vi "build token URI.vi"(8 "error in (no error)":errorcluster, 11 "Oauth2.Google in":refnum<class "Oauth2.Google.lvclass">) -> (0 "error out":errorcluster, 1 "Headers":cluster{"header":string, "value":string}[](array[cluster]), 2 "Token Request URI":string, 3 "Oauth2.Google":refnum<class "Oauth2.Google.lvclass">)   [LabVIEW 2013, in "Oauth2.Google.lvclass"]
uses:
  Oauth2.Google.lvclass
  OAuthToken/OAuth2 Token Element -- enum.ctl
  Oauth2.Google.lvclass/Oauth2.Google.ctl
  <vilib>/LabVIEW Open Source Project/OpenURI/uri/URI.lvclass
  OAuthToken/OAuthAccessToken.lvclass
  Oauth2/Oauth2.lvclass
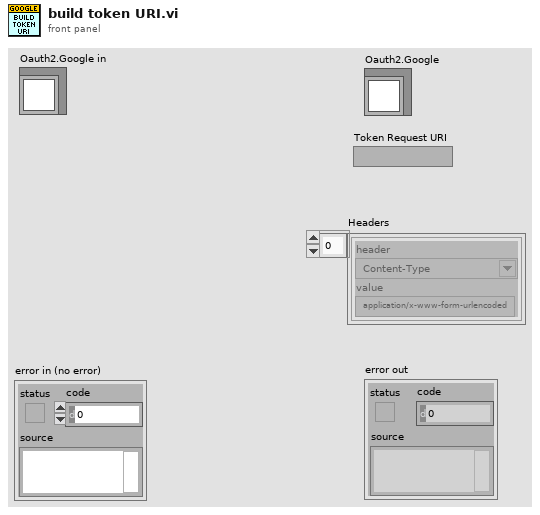
[diagram p1: front panel]
types:
  T1 = typedef "OAuthAccessToken.lvclass/OAuth2 Token Element -- enum.ctl" = enum16{"client_id", "client_secret", "response_type", "scope", "redirect_uri", "error", "error_description", "error_uri", "grant_type", "code", "access_token", "token_type", "expires_in", "username", "password", "refresh_token", "code_challenge", "code_challenge_method", "reverse_proxy_uri", "endpoint element"}
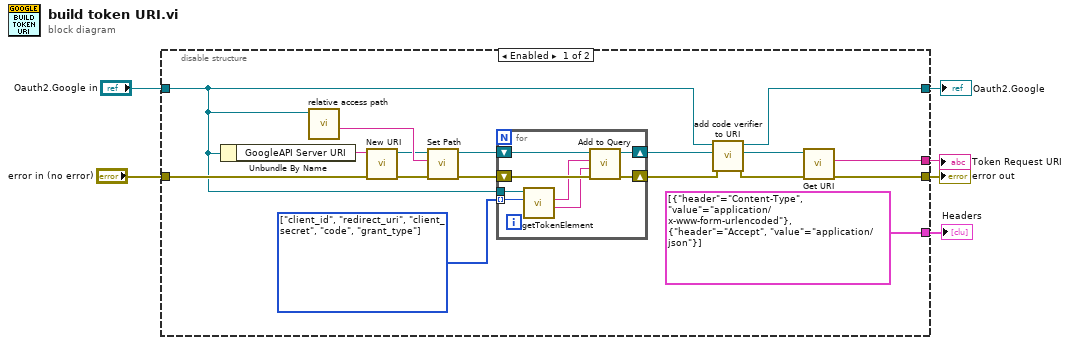
[diagram p0: block diagram]
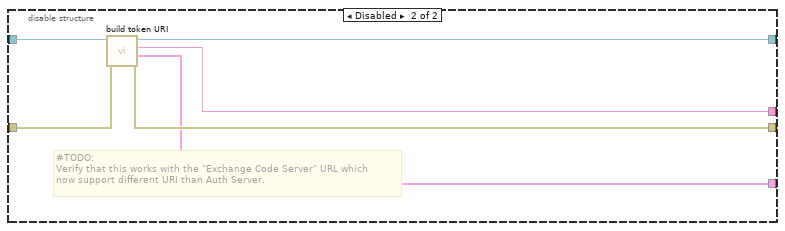
[diagram p2: hidden frame]
diagram:
  n1 = disable-structure shown="Enabled" {
    disable-tunnel: [w18 w35] -> w6
    disable-tunnel: "Oauth2.Google in" -> [w8 w37]
    disable-tunnel: [w16 w33] -> w4
    disable-tunnel: "error in (no error)" -> [w15 w34]
    disable-tunnel: [w7 w36] -> w2
    disable-tunnel: [cluster{"header":string, "value":string}[] [{"header"="Content-Type", "value"="application/x-www-form-urlencoded"}, {"header"="Accept", "value"="application/json"}] ("Headers") w32] -> w1
    frame Enabled {
      w17 = T1[] [enum."client_id", enum."redirect_uri", enum."client_secret", enum."code", enum."grant_type"] items=["client_id", "client_secret", "response_type", "scope", "redirect_uri", "error", "error_description", "error_uri", "grant_type", "code", "access_token", "token_type", "expires_in", "username", "password", "refresh_token", "code_challenge", "code_challenge_method", "reverse_proxy_uri", "endpoint element"]
      n2 = Unbundle By Name(w8) -> ("GoogleAPI Server URI"=w20:string)
      n3 = call-dynamic "relative access path.vi"("Oauth2.Google"=w8) -> ("Token Access Path"=w23:string)  [unwired: 9 in, 1 out]
      n4 = call <vilib>:"New URI.vi"("error in (no error)"=w15, "URI"=w20) -> ("error out"=w14:errorcluster, "URI"=w19:refnum<class "URI.lvclass">)  [unwired: 8 in]
      n5 = call <vilib>:"Set Path.vi"("error in (no error)"=w14, "path"=w23, "URI in"=w19) -> ("error out"=w21:errorcluster, "URI out"=w22:refnum<class "URI.lvclass">)  [unwired: 7 in]
      n6 = for {
        shift-right: [w30] -> w12
        shift-left: w22 -> [w31]
        shift-right: [w28] -> w10
        shift-left: w21 -> [w29]
        tunnel: w8 -> [w27]
        tunnel: w17 -> [w24] mode=indexing
        n7 = call "getTokenElement.vi"("Token element"=w24, "Oauth2 in"=w27) -> ("Value"=w25:string, "Key"=w26:string)  [unwired: 5 in, 3 out]
        n8 = call <vilib>:"Add to Query.vi"("error in (no error)"=w29, "value"=w25, "key"=w26, "URI in"=w31) -> ("error out"=w28:errorcluster, "URI out"=w30:refnum<class "URI.lvclass">)  [unwired: 6 in]
      }
      n9 = call "add code verifier to URI.vi"("error in (no error)"=w10, "URI in"=w12, "Oauth2 in"=w8) -> ("error out"=w9:errorcluster, "URI out"=w11:refnum<class "URI.lvclass">, "Oauth2 out"=w7:refnum<class "Oauth2.Google.lvclass">)  [unwired: 6 in]
      n10 = call <vilib>:"Get URI.vi"("error in (no error)"=w9, "URI in"=w11) -> ("error out"=w16:errorcluster, "URI String"=w18:string)  [unwired: 7 in, 1 out]
    }
    frame Disabled {
      # "#TODO: \nVerify that this works with the \"Exchange Code Server\" URL which\nnow support different URI than Auth Server."
      n11 = call-parent "build token URI.vi"("error in (no error)"=w34, "Oauth2 in"=w37) -> ("error out"=w33:errorcluster, "Headers"=w32:cluster{"header":string, "value":string}[], "Token Request URI"=w35:string, "Oauth2"=w36:refnum<class "Oauth2.Google.lvclass">)  [unwired: 6 in]
    }
  }
  "Token Request URI" <- w6
  "Oauth2.Google" <- w2
  "error out" <- w4
  "Headers" <- w1
